vi "Test Suite Name for Parametrized Test Cases.vi"(11 "Test Case In":refnum<class "Parameterized Test Case Test.lvclass">) -> (0 "error out":errorcluster, 3 "Test Case Out":refnum<class "Parameterized Test Case Test.lvclass">)   [LabVIEW 2020, in "Parameterized Test Case Test.lvclass"]
uses:
  Parameterized Test Case Test.lvclass
  C:/Program Files (x86)/National Instruments/LabVIEW 2020/vi.lib/Astemes/LUnit/Test Case.lvclass
  source/Parametrized Test Case Test Double/Parametrized Test Case Test Double.lvclass
  <vilib>/Astemes/LUnit/Test Case.lvclass/Test Case.ctl
  bba278e5-7b64-463b-bdc4-4e2659b25cb4.vi
  <vilib>/Astemes/LUnit/Append Pass Result.vi
  <vilib>/Astemes/LUnit/Append Fail Result.vi
  <vilib>/Astemes/LUnit/Describe Comparison.vi
  <vilib>/Astemes/LUnit/Compare Variants.vi
  <vilib>/Astemes/LUnit/Run In UI.vi
  <vilib>/Utility/error.llb/Clear Errors.vi
  <vilib>/Astemes/LUnit/Describe Variant.vi
  <vilib>/Astemes/LUnit/Test Suite.lvclass
  Parameterized Test Case Test.lvclass/Parameterized Test Case Test.ctl
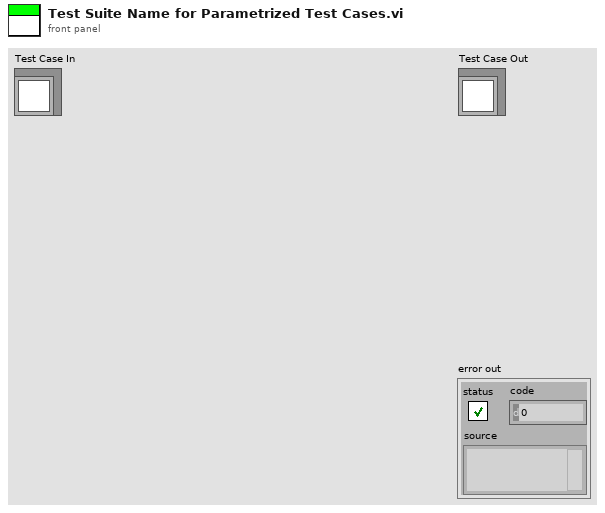
[diagram p1: front panel]
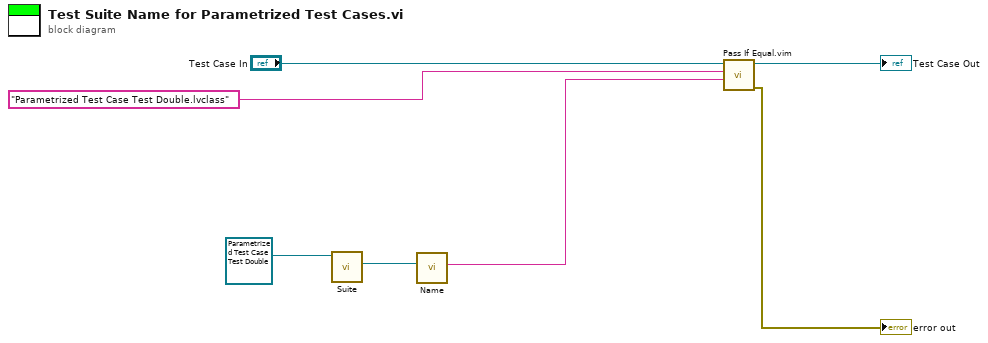
[diagram p0: block diagram]
diagram:
  n1 = call-dynamic "Suite.vi"("Parameterized Test Case In"=refnum<class "Parametrized Test Case Test Double.lvclass"> refnum ("Parametrized Test Case Test Double.lvclass")) -> ("LUnit Test Suite Out"=w2:refnum<class "Test Suite.lvclass">)  [unwired: 8 in, 2 out]
  n2 = call-dynamic "Name.vi"("LUnit Test Suite in"=w2) -> ("Name"=w1:string)  [unwired: 8 in, 2 out]
  n3 = call "Pass If Equal.vim"("Actual"=w1, "Expected"="Parametrized Test Case Test Double.lvclass" ("String"), "LUnit Test Case In"="Test Case In") -> ("error out"=→"error out":errorcluster, "LUnit Test Case Out"=→"Test Case Out":refnum<class "Parameterized Test Case Test.lvclass">)  [unwired: 7 in]
